vi "Load x-y data from File.vi"(4 "file path":path) -> (0 "Y-Array":sgl[](array[numeric]), 1 "X-Array":sgl[](array[numeric]))   [LabVIEW 2021]
uses:
  <vilib>/Utility/file.llb/Read From Spreadsheet File (DBL).vi
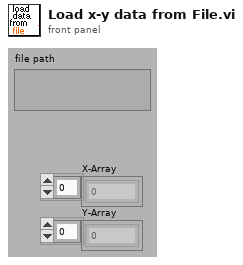
[diagram p1: front panel]
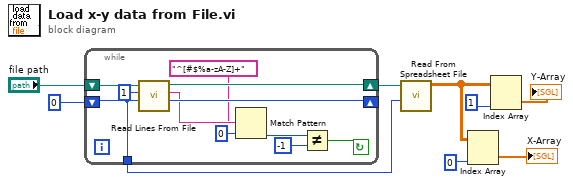
[diagram p0: block diagram]
diagram:
  n1 = while {
    tunnel: [w10] -> w8
    shift-left: 0 ("mark after read (chars.)") -> [w10]
    shift-right: [w17] -> _
    shift-left: "file path" -> [w20]
    shift-right: [w19] -> w7
    stop <- w13 continue-if-true
    n2 = call <vilib>:"Read Lines From File.vi"("file path (dialog if empty)"=w20, "number of lines (all:-1)"=1, "start of read offset (chars.:0)"=w10) -> ("new file path (Not A Path if cancelled)"=w19:path, "line string"=w16:string, "mark after read (chars.)"=w17:i32)  [unwired: 3 in, 1 out]
    n3 = Match Pattern(string=w16, regular expression="^[#$%a-zA-Z]+", offset (0)=0) -> (offset past match=w12:i32)  [unwired: 3 out]
    n4 = Not Equal?(x=w12, y=-1) -> (x != y?=w13:bool)
  }
  n5 = call-poly <vilib>:"Read From Spreadsheet File.vi"("start of read offset (chars.:0)"=w8, "file path (dialog if empty)"=w7) -> ("all rows"=w3:dbl[][])  [unwired: 5 in, 4 out]
  n6 = Index Array(array=w3, index (col)=0) -> (element=→"X-Array":dbl[])  [unwired: 1 in]
  n7 = Index Array(array=w3, index (col)=1) -> (element=→"Y-Array":dbl[])  [unwired: 1 in]
